vi "RD Digital In Trigger Slope Set.vi"(8 "error in (no error)":errorcluster caption="错误输入（无错误）", 10 "slope":i32, 11 "handle":u64) -> (0 "error out":errorcluster caption="错误输出", 2 "function return":i32, 3 "handle out":u64)   [LabVIEW 2018, in "InstrumentsPlayground.lvlib"]
doc: "CLIFFAPI int CliffDigitalInTriggerSlopeSet(FT_HANDLE handle,CLIFFTriggerSlope slope);\nwhen trigger mode ！= digital In trigger\nslope: 0:raising, 1:falling, 2:either"
uses:
  InstrumentsPlayground.lvlib
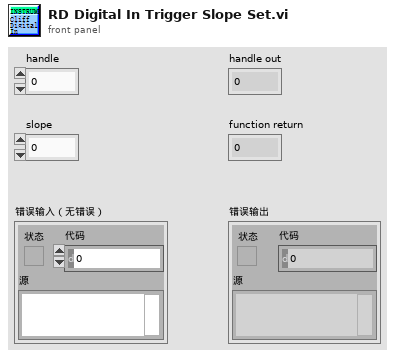
[diagram p1: front panel]
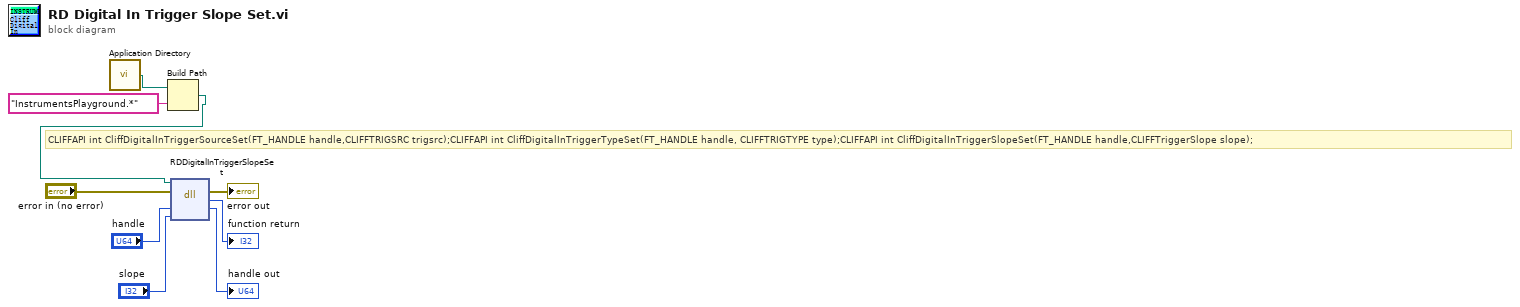
[diagram p0: block diagram]
diagram:
  # "CLIFFAPI int CliffDigitalInTriggerSourceSet(FT_HANDLE handle,CLIFFTRIGSRC trigsrc);CLIFFAPI int CliffDigitalInTriggerTypeSet(FT_HANDLE handle, CLIFFTRIGTYPE type);CLIFFAPI int CliffDigitalInTriggerSlopeSet(FT_HANDLE handle,CLIFFTriggerSlope slope);"
  n1 = call <vilib>:"Application Directory.vi"() -> ("Application Directory"=w2:path)
  n2 = Build Path(base path=w2, name or relative path="InstrumentsPlayground.*" ("名称或相对路径")) -> (appended path=w1:path)
  n3 = dll-call lib="E:/work/YZCourse_Xtext/Cliff/API/LabVIEW lib/InstrumentsPlayground.*" fn="RDDigitalInTriggerSlopeSet"(path in=w1, error in="error in (no error)", "handle"="handle", "slope"="slope") -> (error out=→"error out":errorcluster, "返回类型"=→"function return":i32, "handle"=→"handle out":u32)  [unwired: 2 in, 1 out]
